vi "Score_DB.vi"(5 "Score":u64, 7 "error in (no error)":errorcluster, 8 "Enum":enum16{"Read", "Write"}(ring)) -> (0 "error out":errorcluster, 3 "max score":i32)   [LabVIEW 2010]
uses:
  <vilib>/addons/database/NI_Database_API.lvlib
  <vilib>/addons/database/Connection.llb/DB Tools Open Connec (String).vi
  <vilib>/addons/database/Connection.llb/Conn Execute.vi
  <vilib>/addons/database/Recordset.llb/Rec Fetch Recordset Data (R).vi
  <vilib>/addons/database/Recordset.llb/Rec Destroy - Connection.vi
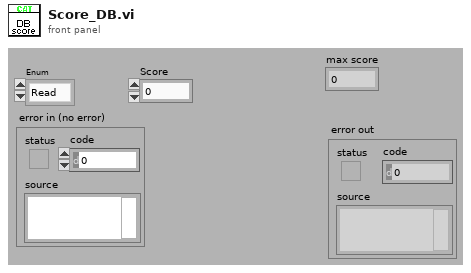
[diagram p1: front panel]
types:
  T1 = typedef "NI_Database_API.lvlib/Conn ObjectReference.ctl" = refnum<k1>
  T2 = typedef "NI_Database_API.lvlib/Rec ObjectReference.ctl" = refnum<k1>
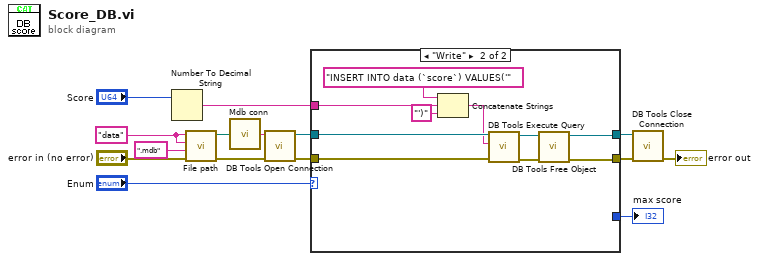
[diagram p0: block diagram]
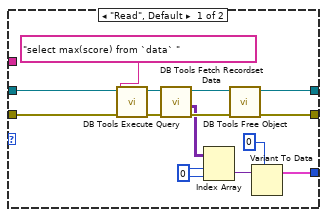
[diagram p2: hidden frame]
diagram:
  w5 = "data" ("folder name")
  n1 = Number To Decimal String(number="Score") -> (decimal integer string=w2:string)  [unwired: 1 in]
  n2 = call "File path.vi"("folder name"=w5, "file name"=w5, "pattern"=".mdb", "error in (no error)"="error in (no error)") -> ("build path"=w6:path, "error out"=w8:errorcluster)  [unwired: 3 out]
  n3 = call "Mdb conn.vi"("input 1"=w6) -> ("resulting string"=w15:string)
  n4 = call-poly <vilib>:"DB Tools Open Connection.vi"("error in (no error)"=w8, "connection information"=w15) -> ("error out"=w13:errorcluster, "connection reference"=w14:T1)  [unwired: 6 in]
  n5 = case shown="\"Write\"" "Enum" {
    tunnel: w14 -> [w29 w39]
    tunnel: w13 -> [w28 w38]
    tunnel: [w23 w35] -> w11
    tunnel: [w22 w34] -> w10
    tunnel: w2 -> [_ w31]
    tunnel: [w18 _] -> w3
    frame "Read", Default {
      w17 = 0 ("index (row)")
      n6 = call-poly <vilib>:"DB Tools Execute Query.vi"("error in (no error)"=w28, "SQL query"="select max(score) from `data` ", "connection reference"=w29) -> ("error out"=w26:errorcluster, "recordset reference"=w27:T2)  [unwired: 5 in]
      n7 = call-poly <vilib>:"DB Tools Fetch Recordset Data.vi"("error in (no error)"=w26, "recordset reference"=w27) -> ("error out"=w25:errorcluster, "recordset data"=w20:variant[][], "recordset reference out"=w24:T2)  [unwired: 3 in]
      n8 = Index Array(array=w20, index (row)=w17, index (col)=w17) -> (element=w19:variant)
      n9 = call-poly <vilib>:"DB Tools Free Object.vi"("error in (no error)"=w25, "recordset reference"=w24) -> ("error out"=w22:errorcluster, "connection reference"=w23:T1)  [unwired: 8 in]
      n10 = Variant To Data(Variant=w19, type=0) -> (data=w18:cluster{})  [unwired: 1 in, 1 out]
    }
    frame "Write" {
      n11 = Concatenate Strings("INSERT INTO data (`score`) VALUES('" ("SQL query"), w31, "')" ("string")) -> (w32:string)
      n12 = call-poly <vilib>:"DB Tools Execute Query.vi"("error in (no error)"=w38, "SQL query"=w32, "connection reference"=w39) -> ("error out"=w36:errorcluster, "recordset reference"=w37:T2)  [unwired: 5 in]
      n13 = call-poly <vilib>:"DB Tools Free Object.vi"("error in (no error)"=w36, "recordset reference"=w37) -> ("error out"=w34:errorcluster, "connection reference"=w35:T1)  [unwired: 8 in]
    }
  }
  "max score" <- w3
  n14 = call <vilib>:"DB Tools Close Connection.vi"("error in (no error)"=w10, "connection reference"=w11) -> ("error out"=→"error out":errorcluster)  [unwired: 5 in]
